vi "Delay Signal.vi"() -> ()   [LabVIEW 2023]
doc: "Demonstrates how to use the DFD Integer Delay VI to delay signals by a specified integer number of sample intervals.\n\nComplete the following steps to use this VI.\n1) Run the VI.\n2) Change the number of delayed samples in the <B>Delay</B> input and run the VI again.\n3) Observe the Signals graph to see if the Delayed Signal plot shifts to the right side of the Original Signal plot by the specified number of samples."
uses:
  <vilib>/addons/Digital Filter Design/Process.llb/DFD Integer Delay (Array).vi
  <vilib>/Analysis/NI_AALBase.lvlib
  <vilib>/addons/Digital Filter Design/NI_DigFilterLicensed.lvlib
panel:
  out "Error Message":string
  out "Signals":dbl[][](graph)
  in  "Delay":i32=5
  # "Select Help>>Show Context Help and move the cursor over the VI icon for more information."
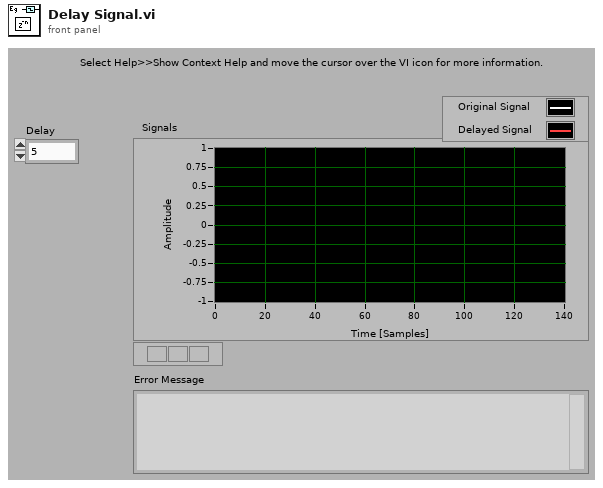
[diagram p1: front panel]
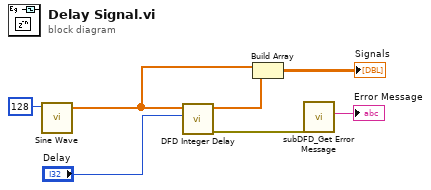
[diagram p0: block diagram]
diagram:
  n1 = call <vilib>:"Sine Wave.vi"("samples"=128) -> ("sine wave"=w5:dbl[])  [unwired: 4 in, 2 out]
  n2 = call-poly <vilib>:"DFD Integer Delay.vi"("delay"="Delay", "signal in"=w5) -> ("error out"=w1:errorcluster, "signal out"=w6:dbl[])  [unwired: 2 in, 6 out]
  n3 = Build Array(w5, w6) -> (→"Signals":dbl[][])
  n4 = call <vilib>:"subDFD_Get Error Message.vi"("error in (no error)"=w1) -> ("Error Message"=→"Error Message":string)  [unwired: 10 out]
